vi "execution class name.vi"(8 "error in":errorcluster, 11 "E2E Tag Exchange configuration in":refnum<class "E2E Tag Exchange configuration.lvclass">) -> (0 "error out":errorcluster, 2 "class name":string, 3 "E2E Tag Exchange configuration out":refnum<class "E2E Tag Exchange configuration.lvclass">)   [LabVIEW 2015, in "E2E Tag Exchange configuration.lvclass"]
doc: "Provides an interface for determining the module runtime class associated with this module configuration. This class name can then be used to dynamically load or locate the runtime class for initialization purposes."
uses:
  E2E Tag Exchange configuration.lvclass
  E2E Tag Exchange configuration.lvclass/E2E Tag Exchange configuration.ctl
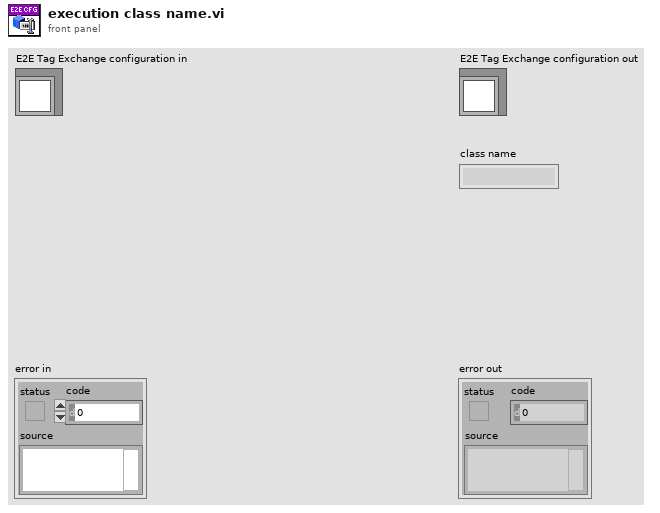
[diagram p1: front panel]
types:
  T1 = typedef "E2E Tag Exchange configuration.lvclass/Runtime Implementation.ctl" = enum16{"RT FIFO", "UDP"}
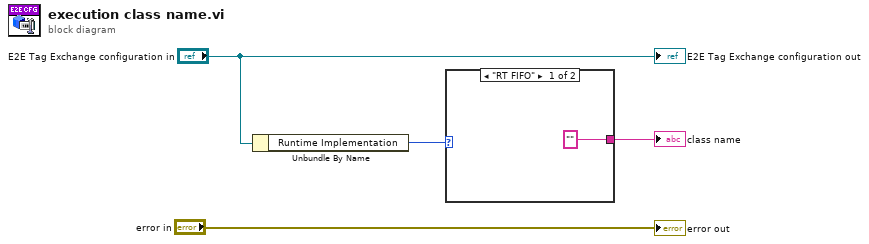
[diagram p0: block diagram]
diagram:
  n1 = Unbundle By Name("E2E Tag Exchange configuration in") -> ("Runtime Implementation"=w3:T1)
  n2 = case shown="\"RT FIFO\"" w3 {
    tunnel: ["" _] -> w1
    frame "RT FIFO" {
    }
    frame "UDP" {
    }
  }
  "class name" <- w1
  "error out" <- "error in"
  "E2E Tag Exchange configuration out" <- "E2E Tag Exchange configuration in"
